vi "daqio_Connect_User.vi"(6 "daq.io API base":string="http://dashboard.daq.io/api/v1", 8 "error in (no error)":errorcluster, 10 "Credentials":T3) -> (0 "error out":errorcluster, 2 "logged in?":bool, 3 "daq.io type":T1={"daq.io ref"=refnum, "daq.io API Base"="http://dashboard.daq.io/api/v1", "Device Type Key"="", "Device Key"="", "Account ID"=""})   [LabVIEW 2013, in "daqio minimal.lvlib"]
doc: "This VI connects the current user to the daq.io cloud connection."
uses:
  daqio minimal.lvlib
  _typedefs/daqio-Credentials.ctl
  _typedefs/daqio-Type.ctl
  <vilib>/httpClient/ClientHandle.ctl
  _typedefs/daqio-Credentials-FGV.ctl
  <vilib>/httpClient/LabVIEWHTTPClient.lvlib
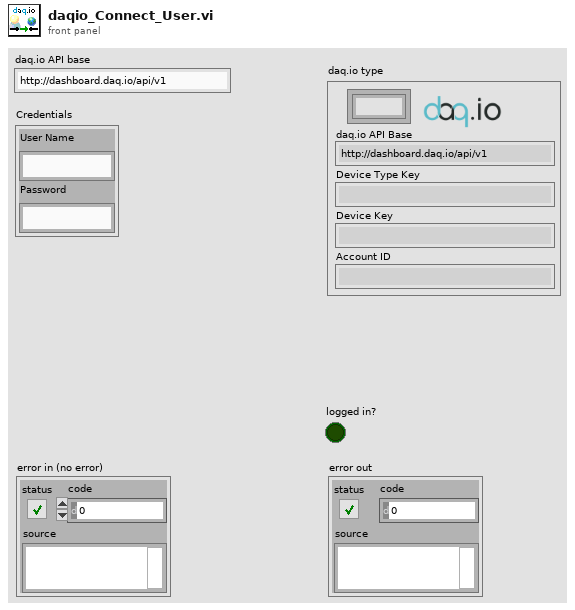
[diagram p1: front panel]
types:
  T1 = typedef "daqio minimal.lvlib/daqio-Type.ctl" = cluster{"daq.io ref":T2, "daq.io API Base":string, "Device Type Key":string, "Device Key":string, "Account ID":string}
  T2 = typedef "LabVIEWHTTPClient.lvlib/ClientHandle.ctl" = refnum<k1>
  T3 = typedef "daqio minimal.lvlib/daqio-Credentials.ctl" = cluster{"User Name":string, "Password":string}
  T4 = typedef "daqio minimal.lvlib/daqio-Credentials-FGV.ctl" = enum16{"Generate", "Read"}
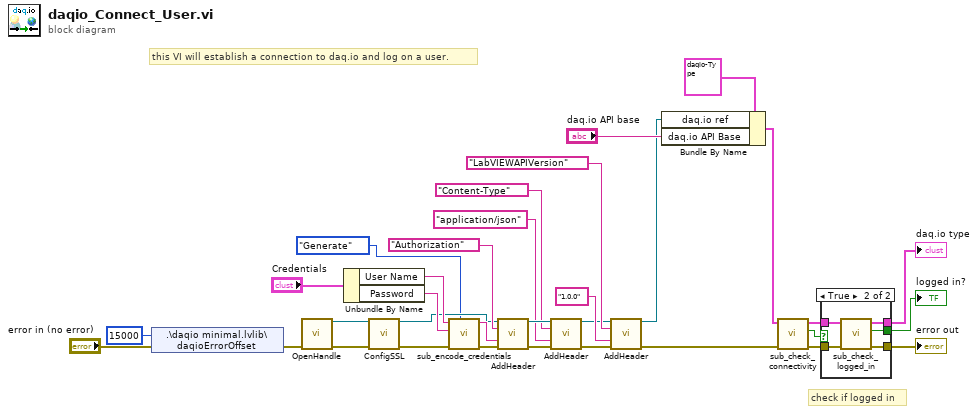
[diagram p0: block diagram]
diagram:
  # "this VI will establish a connection to daq.io and log on a user."
  # "check if logged in"
  n1 = shared-variable ".\\daqio minimal.lvlib\\daqioErrorOffset"(15000 ("daqioErrorOffset"), error in="error in (no error)") -> (error out=w6:errorcluster)
  n2 = call <vilib>:"OpenHandle.vi"("error in (no error)"=w6) -> ("client handle out"=w3:T2, "error out"=w24:errorcluster)  [unwired: 13 in]
  n3 = Unbundle By Name("Credentials") -> ("User Name"=w23:string, "Password"=w22:string)
  n4 = call <vilib>:"ConfigSSL.vi"("client handle"=w3, "error in (no error)"=w24) -> ("client handle out"=w18:T2, "error out"=w19:errorcluster)  [unwired: 12 in]
  n5 = call "sub_encode_credentials.vi"("Command"=daqio-Credentials-FGV."Generate", "error in (no error)"=w19, "Password"=w22, "User Name"=w23) -> ("error out"=w20:errorcluster, "Credentials"=w21:string)  [unwired: 5 in, 1 out]
  n6 = call <vilib>:"AddHeader.vi"("client handle"=w18, "header"="Authorization", "value"=w21, "error in (no error)"=w20) -> ("client handle out"=w31:T2, "error out"=w30:errorcluster)  [unwired: 10 in]
  n7 = call <vilib>:"AddHeader.vi"("client handle"=w31, "header"="Content-Type", "value"="application/json", "error in (no error)"=w30) -> ("client handle out"=w25:T2, "error out"=w26:errorcluster)  [unwired: 10 in]
  n8 = call <vilib>:"AddHeader.vi"("client handle"=w25, "header"="LabVIEWAPIVersion", "value"="1.0.0", "error in (no error)"=w26) -> ("client handle out"=w2:T2, "error out"=w9:errorcluster)  [unwired: 10 in]
  n9 = Bundle By Name(cluster=T1 {"daq.io ref"=refnum, "daq.io API Base"="http://dashboard.daq.io/api/v1", "Device Type Key"="", "Device Key"="", "Account ID"=""} ("daq.io type 2"), "daq.io ref"=w2, "daq.io API Base"="daq.io API base") -> (w8:T1)
  n10 = call "sub_check_connectivity.vi"("error in (no error)"=w9, "daq.io type in"=w8) -> ("error out"=w10:errorcluster, "connected"=w7:bool, "daq.io type out"=w11:T1)  [unwired: 7 in]
  n11 = case shown="True" w7 {
    selector: w7 -> [w36 _]
    tunnel: [w34 w41] -> w14
    tunnel: [w36 w40] -> w13
    tunnel: [w35 w39] -> w12
    tunnel: w11 -> [w34 w38]
    tunnel: w10 -> [w35 w37]
    frame False {
    }
    frame True {
      n12 = call "sub_check_logged_in.vi"("error in (no error)"=w37, "daq.io type in"=w38) -> ("error out"=w39:errorcluster, "logged in?"=w40:bool, "daq.io type out"=w41:T1)  [unwired: 7 in]
    }
  }
  "error out" <- w12
  "daq.io type" <- w14
  "logged in?" <- w13
